vi "Initialise Deployable.vi"(8 "Hotspots":refnum<class "Vector 2D.lvclass">[](array[class]), 9 "Textures":string[](array[string]), 10 "Player Type":T1, 11 "Deployable in":refnum<class "Deployable.lvclass">) -> (3 "Deployable out":refnum<class "Deployable.lvclass">)   [LabVIEW 2021, in "Deployable.lvclass"]
uses:
  Deployable.lvclass
  C:/dev/LabVIEW/LabMelee/Source/Application Specific/Element/Element.lvclass
  Re-use Libraries/Vector 2D/Vector 2D.lvclass
  Element/Player Type.ctl
  Element/Element.lvclass/Element.ctl
  Deployable.lvclass/Deployable.ctl
  Element/Element.lvclass
  Motion/Motion.lvclass
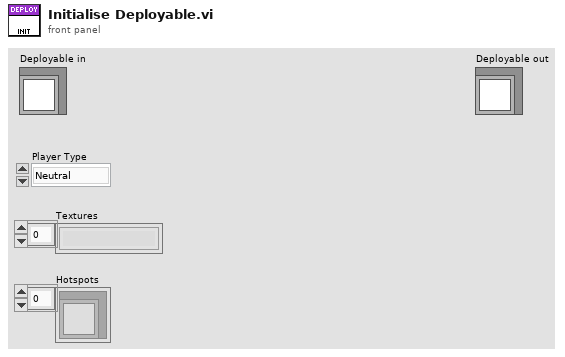
[diagram p1: front panel]
types:
  T1 = typedef "Element.lvclass/Player Type.ctl" = enum16{"Neutral", "Player 1", "Player 2"}
  T2 = typedef "Constants.ctl" = cluster{"Colours":cluster{"OK":u32, "Warning":u32, "Error":u32, "Red":u32, "Green":u32, "Blue":u32, "Yellow":u32}, "System":cluster{"Target Frames Second":dbl, "World Size":T3, "Window Size":T3, "Battle Area Size":T3, "Sidebar Width":sgl, "SC2 Frame Rate [Seconds/Frame]":sgl, "Sidebar Player 2 Y Offset":sgl, "Windows Size V2":refnum<class "Vector 2D.lvclass">, "World Size V2":refnum<class "Vector 2D.lvclass">, "Battle Area Size V2":refnum<class "Vector 2D.lvclass">}, "Game":cluster{"Maximum Asteroids":i32, "Max Energy":i32, "Max Crew":i32, "Maximum Stars":i32}}
  T3 = typedef "SDL2 Utility.lvlib/Point (I32).ctl" = cluster{"x":i32, "y":i32}
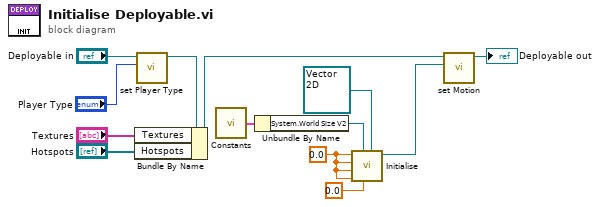
[diagram p0: block diagram]
diagram:
  w8 = sgl 0.0 ("Initial Velocity [m/s]")
  n1 = call "set Player Type.vi"("Player Type"="Player Type", "Element in"="Deployable in") -> ("Element out"=w3:refnum<class "Deployable.lvclass">)  [unwired: 9 in]
  n2 = Bundle By Name(cluster=w3, "Textures"="Textures", "Hotspots"="Hotspots") -> (w11:refnum<class "Deployable.lvclass">)
  n3 = call "Constants.vi"() -> ("Constants"=w6:T2)
  n4 = Unbundle By Name(w6) -> ("System.World Size V2"=w5:refnum<class "Vector 2D.lvclass">)
  n5 = call "Initialise.vi"("Initial Position"=refnum<class "Vector 2D.lvclass"> refnum, "Acceleration [m/s/s]"=sgl 0.0, "Field Size"=w5, "Maximum Velocity [m/s]"=w8, "Turn Rate [deg/s]"=w8, "Initial Heading [deg]"=w8, "Initial Velocity [m/s]"=w8) -> ("Motion out"=w9:refnum<class "Motion.lvclass">)  [unwired: 4 in]
  n6 = call "set Motion.vi"("Motion"=w9, "Element in"=w11) -> ("Element out"=→"Deployable out":refnum<class "Deployable.lvclass">)  [unwired: 9 in]
